vi "Constant_Extension_GroupName.vi"() -> (0 "Group Name String":string="flist")   [LabVIEW 2018]
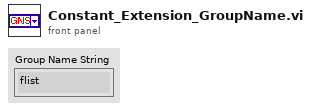
[diagram p1: front panel]
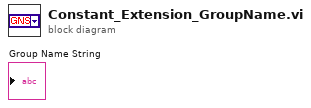
[diagram p0: block diagram]
diagram:
